vi "TagDB-Truncate.vi"(8 "error in (no error)":errorcluster, 10 "with Data?(F)":bool, 11 "TagDB":refnum<k1>) -> (0 "error out":errorcluster, 1 "Data":variant[](array[variant]), 2 "names":string[](array[string]), 3 "TagDB(dup)":refnum<k1>)   [LabVIEW 2017, in "TagDB.lvlib"]
uses:
  TagDB.lvlib
  _Support/Error/_Build Error Cluster.vi
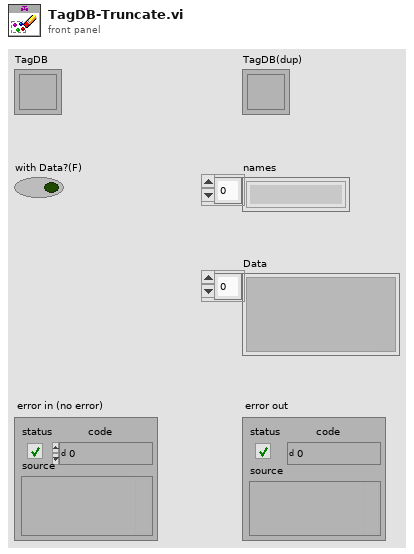
[diagram p1: front panel]
types:
  T1 = typedef "TagDB.lvlib/tagdb-data.ctl" = cluster{"tag-map":variant, "timestamp-map":variant, "namecacher-map":variant, "DataTypeCacher-map":variant, "Tag Adding Lock?":bool, "Global Change Timestamp":timestamp, "Item Change Timestamp":timestamp, "name":string, "Global Change Flag":u64, "Item Change Flag":u64}
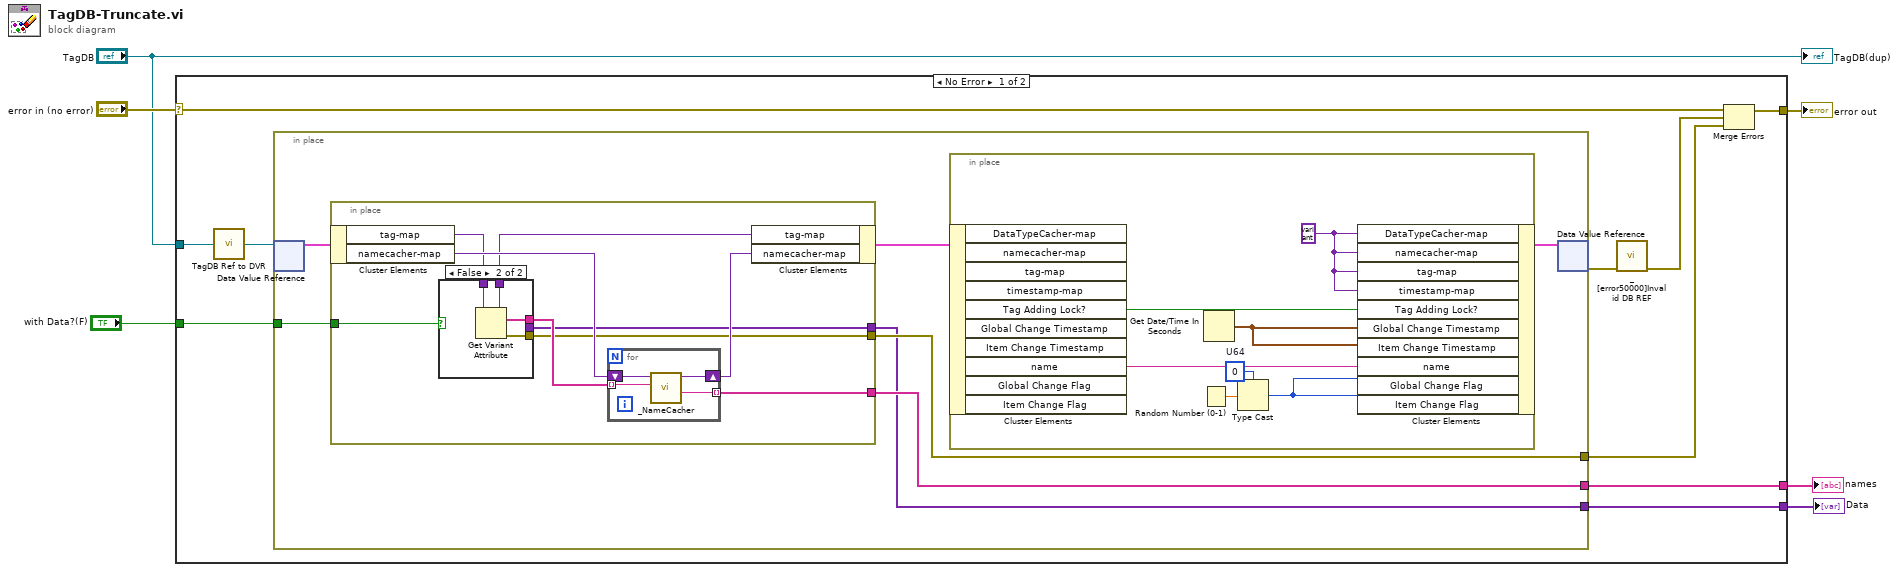
[diagram p0: block diagram]
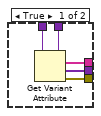
[diagram p2: hidden frame]
diagram:
  n1 = case shown="No Error" "error in (no error)" {
    selector: "error in (no error)" -> [w15 w53]
    tunnel: [w16 w53] -> w5
    tunnel: "TagDB" -> [w13 _]
    tunnel: "with Data?(F)" -> [w10 _]
    tunnel: [w8 _] -> w2
    tunnel: [w7 _] -> w1
    frame No Error {
      n2 = call "TagDB Ref to DVR.vi"("TagDB"=w13) -> ("DVR"=w12:refnum<data-value>)  [unwired: 4 in]
      n3 = in-place "In Place Element Structure" {
        in-place-border: w10 -> [w20]
        in-place-border: [w19] -> w9
        in-place-border: [w18] -> w8
        in-place-border: [w17] -> w7
        n4 = in-place-dvr #1(w12) -> (w22:T1)  [unwired: 1 out]
        n5 = in-place {
          in-place-border: [w33] -> w17
          in-place-border: [w38] -> w18
          in-place-border: [w32] -> w19
          in-place-border: w20 -> [w31]
          n6 = in-place-cluster #2(w22) -> ("tag-map"=w36:variant, "namecacher-map"=w37:variant)
          n7 = case shown="False" w31 {
            tunnel: [w44 w48] -> w39
            tunnel: w36 -> [w43 w47]
            tunnel: [w42 w46] -> w35
            tunnel: [w41 _] -> w33
            tunnel: [w40 w45] -> w32
            frame True {
              n8 = Get Variant Attribute(Variant=w43) -> (duplicate Variant=w42:variant, names=w44:string[], values=w41:variant[], error out=w40:errorcluster)  [unwired: 3 in]
            }
            frame False {
              n9 = Get Variant Attribute(Variant=w47) -> (duplicate Variant=w46:variant, names=w48:string[], error out=w45:errorcluster)  [unwired: 3 in, 1 out]
            }
          }
          n10 = for {
            tunnel: w39 -> [w52] mode=indexing
            tunnel: [w51] -> w38 mode=indexing
            shift-right: [w49] -> w34
            shift-left: w37 -> [w50]
            n11 = call "_NameCacher.vi"("key"=w52, "cacher"=w50) -> ("Raw name"=w51:string, "cacher out"=w49:variant)  [unwired: 7 in, 1 out]
          }
          n12 = in-place-cluster #2("tag-map"=w35, "namecacher-map"=w34) -> (w21:T1)
        }
        n13 = in-place {
          w24 = variant ("DataTypeCacher-map")
          w25 = u64 0  # U64
          n14 = in-place-cluster #3(w21) -> ("Tag Adding Lock?"=w30:bool, "name"=w28:string)  [unwired: 8 out]
          n15 = Random Number (0-1)() -> (number: 0 to 1=w26:dbl)
          n16 = Get Date/Time In Seconds() -> (seconds since 1Jan1904=w29:timestamp)
          n17 = Type Cast(type=w25, x=w26) -> (*(type *) &x=w27:u64)
          n18 = in-place-cluster #3("DataTypeCacher-map"=w24, "namecacher-map"=w24, "tag-map"=w24, "timestamp-map"=w24, "Tag Adding Lock?"=w30, "Global Change Timestamp"=w29, "Item Change Timestamp"=w29, "name"=w28, "Global Change Flag"=w27, "Item Change Flag"=w27) -> (w23:T1)
        }
        n19 = in-place-dvr #1(w23) -> (w14:errorcluster)  [unwired: 1 out]
      }
      n20 = call "_[error50000]Invalid DB REF.vi"("error in (no error)"=w14) -> ("error out"=w11:errorcluster)  [unwired: 10 in]
      n21 = Merge Errors(w15, w11, w9) -> (w16:errorcluster)
    }
    frame Error {
    }
  }
  "error out" <- w5
  "names" <- w2
  "Data" <- w1
  "TagDB(dup)" <- "TagDB"
